vi "ToSignalType.vi"(10 "state":string, 11 "command":T1) -> (3 "Signal":T2)   [LabVIEW 2016]
doc: "Changes between enums - data command enum and signal type enum"
uses:
  SignalType.ctl
  data_command_enum.ctl
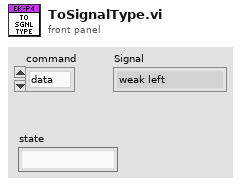
[diagram p1: front panel]
types:
  T1 = typedef "data_command_enum.ctl" = enum16{"data", "display", "quit", "save", "filepath", "weak left", "state", "weak right", "strong left", "strong right", "stopRecording", "close", "sid"}
  T2 = typedef "SignalType.ctl" = enum16{"weak left", "weak right", "strong left", "strong right"}
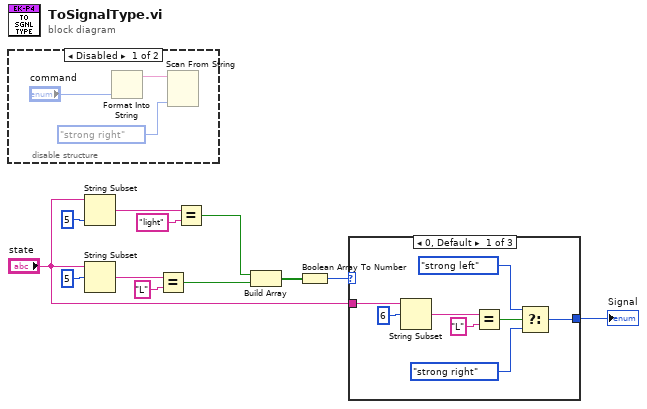
[diagram p0: block diagram]
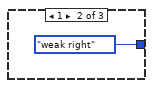
[diagram p3: hidden frame]
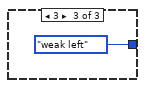
[diagram p4: hidden frame]
diagram:
  n1 = disable-structure shown="Disabled" {
    frame Disabled {
      n2 = Format Into String("command") -> (resulting string=w14:string)  [unwired: 3 in, 1 out]
      n3 = Scan From String(input string=w14, default 1=SignalType."strong right" ("Signal")) -> ()  [unwired: 4 in, 3 out]
    }
    frame Enabled {
    }
  }
  n4 = String Subset(string="state", length (rest)=5 ("length (rest)")) -> (substring=w11:string)  [unwired: 1 in]
  n5 = String Subset(string="state", offset (0)=5) -> (substring=w8:string)  [unwired: 1 in]
  n6 = Equal?(x=w8, y="L") -> (x = y?=w5:bool)
  n7 = Equal?(x=w11, y="light") -> (x = y?=w6:bool)
  n8 = Build Array(w6, w5) -> (w4:bool[])
  n9 = Boolean Array To Number(Boolean array=w4) -> (number=w3:u32)
  n10 = case shown="0, Default" w3 {
    tunnel: [w16 SignalType."weak right" ("Signal") SignalType."weak left" ("Signal")] -> w1
    tunnel: "state" -> [w23 _ _]
    frame 0, Default {
      n11 = String Subset(string=w23, offset (0)=6) -> (substring=w20:string)  [unwired: 1 in]
      n12 = Equal?(x=w20, y="L") -> (x = y?=w19:bool)
      n13 = Select(t=SignalType."strong left" ("Signal"), s=w19, f=SignalType."strong right" ("Signal")) -> (s? t:f=w16:T2)
    }
    frame 1 {
    }
    frame 3 {
    }
  }
  "Signal" <- w1
